vi "JOBJ.vi"() -> ()   [LabVIEW 2017]
uses:
  JSONtext.lvlib
panel:
  out "<JSON> 2":string
  out "error out 2":errorcluster
  out "data 3":cluster{"name":string, "A":string}[](array[cluster])
  out "data 2":cluster{"name":string, "A":string, "B":dbl}[](array[cluster])
  out "error out":errorcluster
  out "<JSON>":string
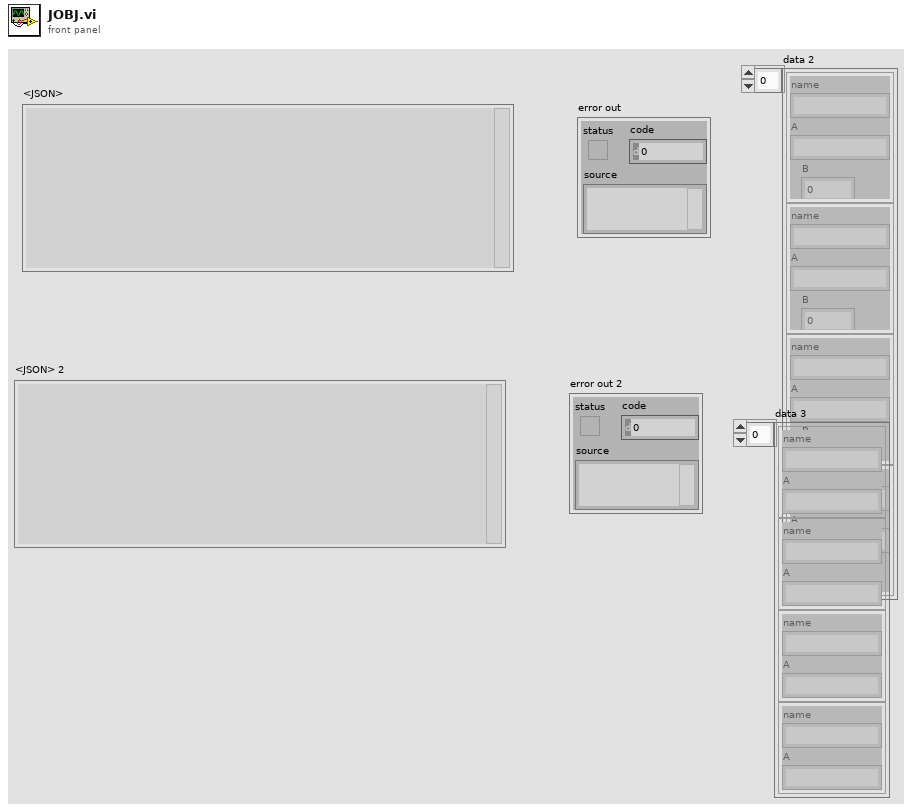
[diagram p1: front panel]
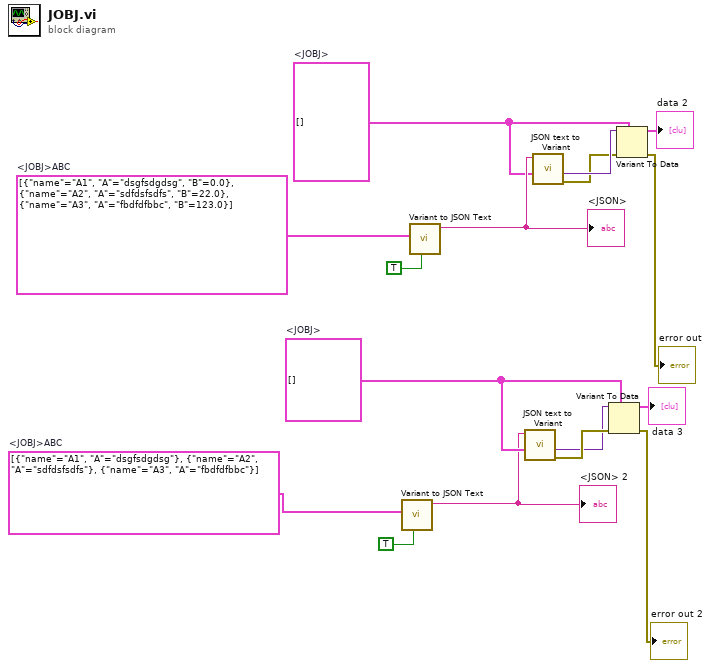
[diagram p0: block diagram]
diagram:
  w7 = cluster{"name":string, "A":string}[] []  # <JOBJ>
  w6 = cluster{"name":string, "A":string}[] [{"name"="A1", "A"="dsgfsdgdsg"}, {"name"="A2", "A"="sdfdsfsdfs"}, {"name"="A3", "A"="fbdfdfbbc"}]  # <JOBJ>ABC
  w10 = cluster{"name":string, "A":string, "B":dbl}[] []  # <JOBJ>
  w11 = cluster{"name":string, "A":string, "B":dbl}[] [{"name"="A1", "A"="dsgfsdgdsg", "B"=0.0}, {"name"="A2", "A"="sdfdsfsdfs", "B"=22.0}, {"name"="A3", "A"="fbdfdfbbc", "B"=123.0}]  # <JOBJ>ABC
  n1 = call "Variant to JSON Text.vi"("Pretty Print?"=TRUE, "Variant"=w6) -> ("<JSON>"=w1:string)  [unwired: 7 in, 2 out]
  "<JSON> 2" <- w1
  n2 = call "Variant to JSON Text.vi"("Pretty Print?"=TRUE, "Variant"=w11) -> ("<JSON>"=w16:string)  [unwired: 7 in, 2 out]
  "<JSON>" <- w16
  n3 = call "JSON text to Variant.vi"("Data Type"=w7, "JSON"=w1) -> ("error out"=w3:errorcluster, "Variant out"=w2:variant)  [unwired: 8 in]
  n4 = call "JSON text to Variant.vi"("Data Type"=w10, "JSON"=w16) -> ("error out"=w14:errorcluster, "Variant out"=w15:variant)  [unwired: 8 in]
  n5 = Variant To Data(error in=w3, type=w7, Variant=w2) -> (data=→"data 3":cluster{"name":string, "A":string}[], error out=→"error out 2":errorcluster)
  n6 = Variant To Data(error in=w14, type=w10, Variant=w15) -> (data=→"data 2":cluster{"name":string, "A":string, "B":dbl}[], error out=→"error out":errorcluster)
